vi "code density mode.vi"(8 "error in (no error)":errorcluster, 11 "IP address":string="192.168.10.17") -> (0 "error out":errorcluster)   [LabVIEW 2017]
panel:
  out "Out":u8 format="%.0x"
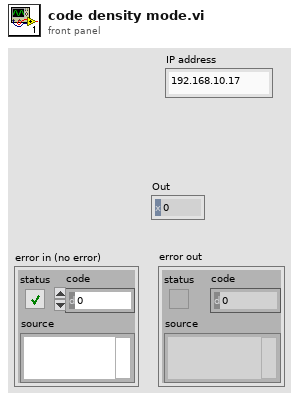
[diagram p1: front panel]
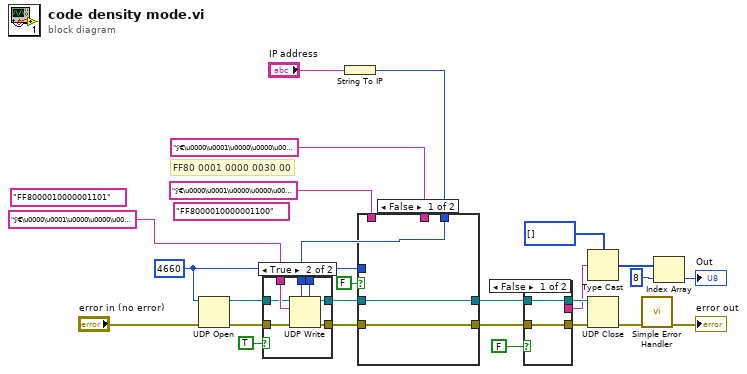
[diagram p0: block diagram]
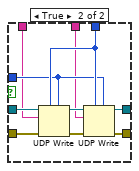
[diagram p2: hidden frame]
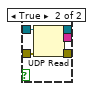
[diagram p4: hidden frame]
diagram:
  (unwired) "FF8000010000001101" ("data in")
  (unwired) "FF8000010000001100" ("data in")
  w10 = u16 4660 ("UDP port")
  # "FF80 0001 0000 0030 00"
  n1 = UDP Open(8:"error in (no error)", 11:w10) -> (port=w7:refnum<k16>, 0:w9:errorcluster)  [unwired: 3 in, 1 out]
  n2 = String To IP(1:"IP address") -> (0:w11:u32)
  n3 = case shown="True" TRUE {
    tunnel: "ÿ€\u0000\u0001\u0000\u0000\u0000\u0011\u0001" ("字符串") -> [_ w34]
    tunnel: w11 -> [_ w33]
    tunnel: w10 -> [_ w32]
    tunnel: w9 -> [w27 w31]
    tunnel: [w27 w30] -> w8
    tunnel: w7 -> [w26 w29]
    tunnel: [w26 w28] -> w6
    frame False {
    }
    frame True {
      n4 = UDP Write(address=w33, port or service name=w32, connection ID=w29, data in=w34, 8:w31) -> (error out=w30:errorcluster, 3:w28:refnum<k16>)  [unwired: 1 in]
    }
  }
  n5 = case shown="False" FALSE {
    tunnel: [w35 w46] -> w24
    tunnel: [w36 w45] -> w22
    tunnel: w11 -> [_ w42]
    tunnel: w10 -> [_ w41]
    tunnel: w8 -> [w36 w40]
    tunnel: w6 -> [w35 w39]
    tunnel: "ÿ€\u0000\u0001\u0000\u0000\u0000\u0010\u0001" ("字符串") -> [_ w38]
    tunnel: "ÿ€\u0000\u0001\u0000\u0000\u0000\u0011\u0000" ("字符串") -> [_ w37]
    frame False {
    }
    frame True {
      n6 = UDP Write(address=w42, port or service name=w41, connection ID=w39, data in=w37, 8:w40) -> (error out=w44:errorcluster, 3:w43:refnum<k16>)  [unwired: 1 in]
      n7 = UDP Write(address=w42, port or service name=w41, connection ID=w43, data in=w38, 8:w44) -> (error out=w45:errorcluster, 3:w46:refnum<k16>)  [unwired: 1 in]
    }
  }
  n8 = case shown="False" FALSE {
    tunnel: w24 -> [w48 w53]
    tunnel: [w48 w52] -> w23
    tunnel: w22 -> [w47 w51]
    tunnel: [w47 w50] -> w21
    tunnel: [_ w49] -> w20
    frame False {
    }
    frame True {
      n9 = UDP Read(connection ID=w53, 8:w51) -> (data out=w49:string, error out=w50:errorcluster, 3:w52:refnum<k16>)  [unwired: 1 in, 3 out]
    }
  }
  n10 = Type Cast(type=u8[] [], x=w20) -> (*(type *) &x=w18:u8[])
  n11 = UDP Close(connection ID=w23, 8:w21) -> (error out=w25:errorcluster)  [unwired: 1 out]
  n12 = call <vilib>:"Simple Error Handler.vi"("error in (no error)"=w25) -> ("error out"=→"error out":errorcluster)  [unwired: 4 in, 4 out]
  n13 = Index Array(array=w18, index=8) -> (element=→"Out":u8)
